vi "Method.vi"(4 "Abs_Waveform.lvclass":refnum<class "Abs_Waveform.lvclass">) -> (1 "Result":refnum<class "Abs_Waveform.lvclass">)   [LabVIEW 2021, in "Increment_WFM.lvclass"]
uses:
  Increment_WFM.lvclass
  Abs_Types/Waveform/Abs_Waveform.lvclass
  C:/TSA/LV_Abstract/Source/Functions/Support/Function/One Terminal/WFM_Numeric/AbsFunc_One Term_WFM_Numeric.lvclass
  C:/Program Files (x86)/National Instruments/LabVIEW 2021/vi.lib/TSA/Abstract Data Classes/Abs_Types/Waveform/Abs_Waveform.lvclass
  Support/Function/One Terminal/WFM_Numeric/AbsFunc_One Term_WFM_Numeric.lvclass/AbsFunc_One Term_WFM_Numeric.ctl
  Support/Function/One Terminal/WFM_Numeric/Properties/Write Abs_Waveform.lvclass.vi
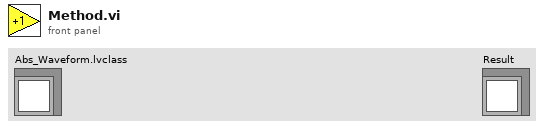
[diagram p1: front panel]
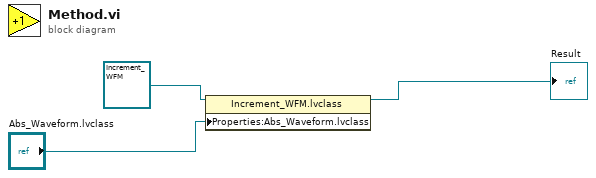
[diagram p0: block diagram]
diagram:
  n1 = property class="Increment_WFM.lvclass"(reference=refnum<class "Increment_WFM.lvclass"> refnum ("Functions.lvlib:Numeric.lvlib:Add_DBL.lvclass"), "Properties:Abs_Waveform.lvclass"="Abs_Waveform.lvclass") -> (reference out=→"Result":refnum<class "Increment_WFM.lvclass">)  [unwired: 1 in, 1 out]
